vi "ROI Selector.vi"() -> ()   [LabVIEW 2012]
panel:
  in  "GridPoints":dbl=5.0
  out "Seting":i32[][](array[numeric])
  in  "Scan Settings":T1={"XStart"=-150000000, "XEnd"=150000000, "XNum"=350, "YStart"=-150000000, "YEnd"=150000000, "YNum"=500, "ZStart"=-30000, "ZEnd"=30000, "ZNum"=30}
  in  "Clear Points":bool
  in  "Section":i32(c297)
  in  "stop":bool
  out "Image":T2(plugin-control)
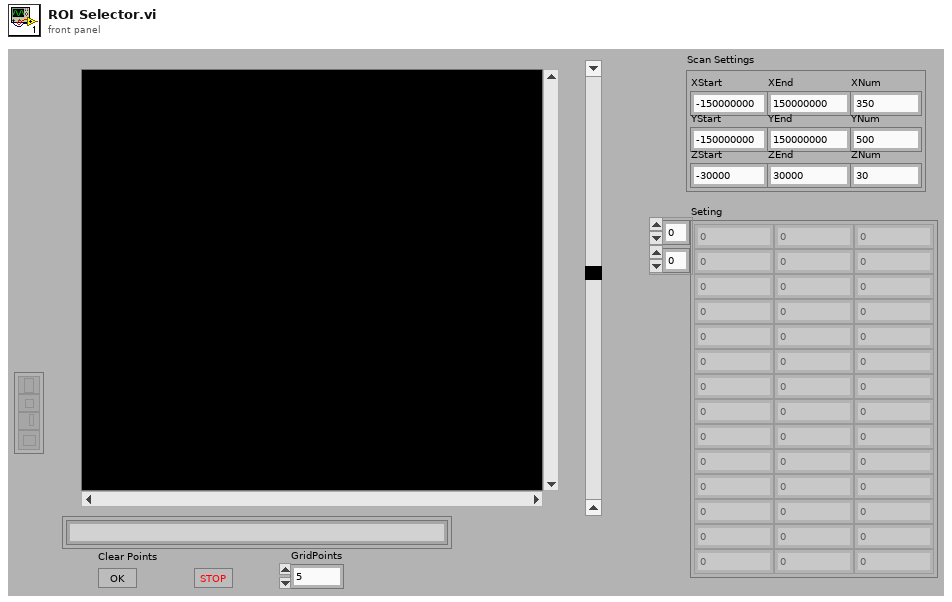
[diagram p1: front panel]
types:
  T1 = cluster{"XStart":i32, "XEnd":i32, "XNum":i32, "YStart":i32, "YEnd":i32, "YNum":i32, "ZStart":i32, "ZEnd":i32, "ZNum":i32}
  T2 = typedef "IMAQ Image.ctl" = refnum<image>
  T3 = cluster{"Global Rectangle":i32[], "Contours":cluster{"Contour Type":u32, "ROI Type":u32, "Points":i32[]}[]}
  T4 = cluster{"Global Rectangle":i32[], "Contours":cluster{"Contour Type":u32, "ROI Type":u32, "Points":i32[]}[]}[]
  T5 = cluster{"Contour Type":u32, "ROI Type":u32, "Points":i32[]}[]
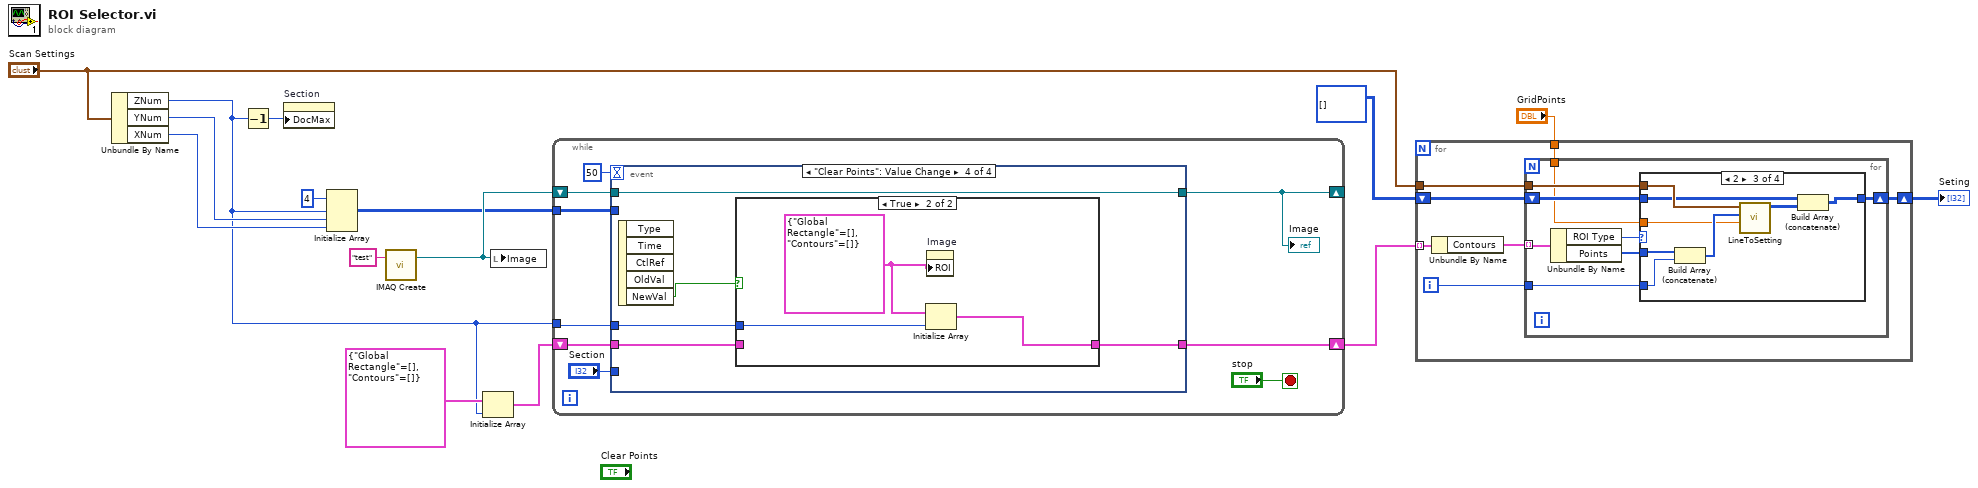
[diagram p0: block diagram]
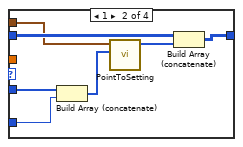
[diagram p3: hidden frame]
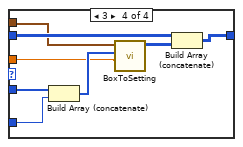
[diagram p4: hidden frame]
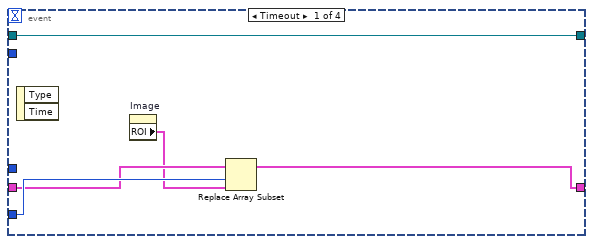
[diagram p5: hidden frame]
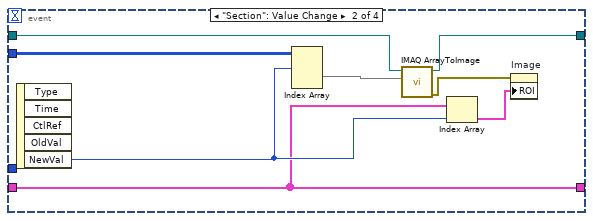
[diagram p6: hidden frame]
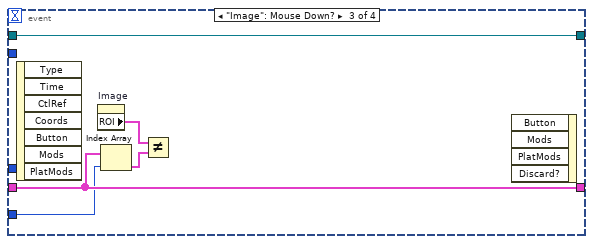
[diagram p7: hidden frame]
diagram:
  n1 = Unbundle By Name("Scan Settings") -> ("ZNum"=w4:i32, "YNum"=w6:i32, "XNum"=w5:i32)
  n2 = Decrement(x=w4) -> (x-1=w8:i32)
  n3 = property on="Section" class="Scroll (strict)"("DocMax"=w8) -> ()  [unwired: 2 in, 2 out]
  n4 = Initialize Array(u8 4 ("element"), w4, w6, w5) -> (w7:u8[][][])
  n5 = call "IMAQ Create"("Image Name"="test") -> ("New Image"=w13:T2)  [unwired: 4 in, 1 out]
  n6 = Initialize Array(T3 {"Global Rectangle"=[], "Contours"=[]} ("ROI"), w4) -> (w11:T4)
  n7 = local write "Image"(w13) -> ()
  n8 = while {
    tunnel: w7 -> [w23]
    shift-right: [w18] -> w10
    shift-left: w11 -> [w21]
    shift-right: [w19] -> _
    shift-left: w13 -> [w20]
    tunnel: w4 -> [w16]
    stop <- "stop" stop-if-true
    n9 = event shown="[3] \"Clear Points\": Value Change" {
      selector: _ -> [_ _ _ _]
      dyn-events: _ -> [_ _ _ _]
      timeout: 50 -> [_ _ _ _]
      tunnel: w23 -> [_ w37 _ _]
      tunnel: w21 -> [w26 w30 w41 w46]
      tunnel: w20 -> [w29 w33 w42 w45]
      tunnel: [w29 w32 w42 w45] -> w19
      tunnel: [w27 w30 w41 w44] -> w18
      tunnel: "Section" -> [w28 _ w40 _]
      tunnel: w16 -> [_ _ _ w43]
      event Timeout {
        n10 = event-data() -> ()  [unwired: 1 in, 2 out]
        n11 = property on="Image" class="ImageControl"() -> ("ROI"=w25:T3)  [unwired: 2 in, 2 out]
        n12 = Replace Array Subset(array=w26, new element=w25, index=w28) -> (w27:T4)
      }
      event "Section": Value Change {
        n13 = event-data() -> ("NewVal"=w31:i32)  [unwired: 1 in, 4 out]
        n14 = Index Array(array=w37, index (dim 0)=w31) -> (element=w36:u8[][])  [unwired: 2 in]
        n15 = call "IMAQ ArrayToImage"("Image Pixels (U8)"=w36, "Image"=w33) -> ("error out"=w34:errorcluster, "Image Out"=w32:T2)  [unwired: 8 in]
        n16 = Index Array(array=w30, index=w31) -> (element=w35:T3)
        n17 = property on="Image" class="ImageControl"(error in=w34, "ROI"=w35) -> ()  [unwired: 1 in, 2 out]
      }
      event "Image": Mouse Down? {
        n18 = event-data() -> ()  [unwired: 1 in, 7 out]
        n19 = property on="Image" class="ImageControl"() -> ("ROI"=w38:T3)  [unwired: 2 in, 2 out]
        n20 = Index Array(array=w41, index=w40) -> (element=w39:T3)
        n21 = Not Equal?(x=w38, y=w39) -> ()  [unwired: 1 out]
        n22 = event-data() -> ()  [unwired: 5 in, 1 out]
      }
      event "Clear Points": Value Change {
        n23 = event-data() -> ("NewVal"=w47:bool)  [unwired: 1 in, 4 out]
        n24 = case shown="True" w47 {
          tunnel: w46 -> [w48 _]
          tunnel: [w48 w51] -> w44
          tunnel: w43 -> [_ w49]
          frame False {
          }
          frame True {
            w50 = T3 {"Global Rectangle"=[], "Contours"=[]} ("ROI")
            n25 = Initialize Array(w50, w49) -> (w51:T4)
            n26 = property on="Image" class="ImageControl"("ROI"=w50) -> ()  [unwired: 2 in, 2 out]
          }
        }
      }
    }
    "Image" <- w19
  }
  n27 = for {
    tunnel: w10 -> [w58] mode=indexing
    shift-right: [w54] -> w2
    shift-left: i32[][] [] -> [w55]
    tunnel: "Scan Settings" -> [w53]
    tunnel: "GridPoints" -> [w52]
    i -> [w56]
    n28 = Unbundle By Name(w58) -> ("Contours"=w57:T5)
    n29 = for {
      tunnel: w57 -> [w66] mode=indexing
      tunnel: w56 -> [w62]
      shift-right: [w61] -> w54
      shift-left: w55 -> [w63]
      tunnel: w53 -> [w60]
      tunnel: w52 -> [w59]
      n30 = Unbundle By Name(w66) -> ("ROI Type"=w65:u32, "Points"=w64:i32[])
      n31 = case shown="2" w65 {
        tunnel: w64 -> [_ w74 w82 w87]
        tunnel: w63 -> [w67 w72 w78 w90]
        tunnel: w62 -> [_ w73 w81 w89]
        tunnel: [w67 w71 w76 w88] -> w61
        tunnel: w60 -> [_ w69 w80 w86]
        tunnel: w59 -> [_ _ w75 w83]
        frame 0, Default {
        }
        frame 1 {
          n32 = Build Array (concatenate)(w74, w73) -> (w68:i32[])
          n33 = call "PointToSetting.vi"("Clicked"=w68, "Scan Settings"=w69) -> ("Setting"=w70:i32[])  [unwired: 9 in]
          n34 = Build Array (concatenate)(w72, w70) -> (w71:i32[][])
        }
        frame 2 {
          n35 = Build Array (concatenate)(w82, w81) -> (w79:i32[])
          n36 = call "LineToSetting.vi"("GridSize"=w75, "Line"=w79, "Scan Settings"=w80) -> ("Settings"=w77:i32[][])  [unwired: 8 in]
          n37 = Build Array (concatenate)(w78, w77) -> (w76:i32[][])
        }
        frame 3 {
          n38 = Build Array (concatenate)(w87, w89) -> (w84:i32[])
          n39 = call "BoxToSetting.vi"("GridSize"=w83, "Line"=w84, "Scan Settings"=w86) -> ("Settings"=w85:i32[][])  [unwired: 8 in]
          n40 = Build Array (concatenate)(w90, w85) -> (w88:i32[][])
        }
      }
    }
  }
  "Seting" <- w2
